vi "Osciloscope teardown.vi"(8 "error in":errorcluster, 11 "Module ID":i32) -> (0 "error out":errorcluster)   [LabVIEW 2020]
doc: "_____\nCreated using DQMH Event Scripter 6.0.0.122."
uses:
  Libraries/Osciloscope/Osciloscope.lvlib
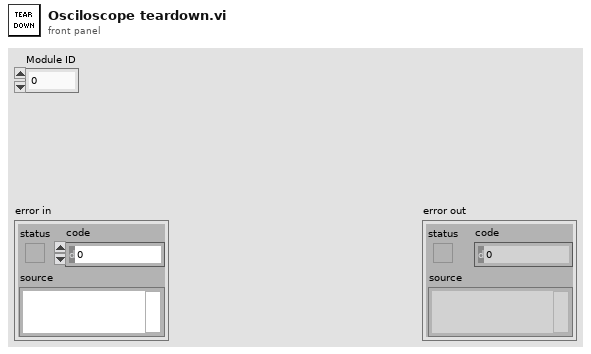
[diagram p1: front panel]
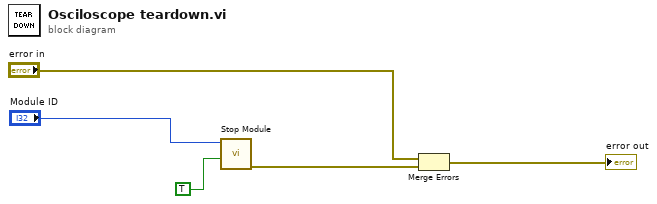
[diagram p0: block diagram]
diagram:
  n1 = call "Stop Module.vi"("Wait for Module to stop? (F)"=TRUE, "Module ID"="Module ID") -> ("error out"=w5:errorcluster)  [unwired: 9 in]
  n2 = Merge Errors("error in", w5) -> (→"error out":errorcluster)
